vi "Check Error Status.vi"(0 "Emergency Stop":bool, 2 "Action (Write)":enum16{"Write", "Read"}(ring), 7 "Error In":errorcluster) -> (8 "Error?":bool)   [LabVIEW 2010]
doc: "This VI is a functional global variable. It checks for errors & remembers if one occurred. This is extremely useful between multiple loops. Be sure to initialize this VI before doing anything else."
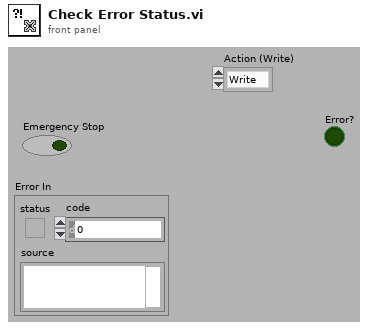
[diagram p1: front panel]
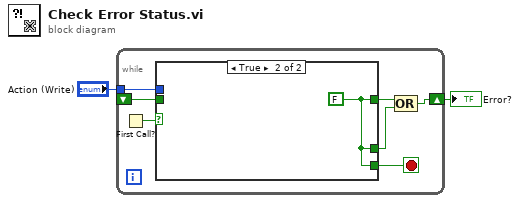
[diagram p0: block diagram]
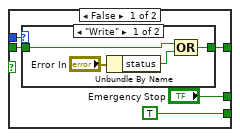
[diagram p2: hidden frame]
diagram:
  n1 = while {
    shift-right: [w5] -> w1
    shift-left: _ -> [w7]
    tunnel: "Action (Write)" -> [w8]
    stop <- w9 stop-if-true
    n2 = First Call?() -> (First Call?: T/F=w3:bool)
    n3 = case shown="TRUE" w3 {
      tunnel: [TRUE w20] -> w9
      tunnel: w8 -> [w13 _]
      tunnel: w7 -> [w12 _]
      tunnel: ["Emergency Stop" w20] -> w6
      tunnel: [w10 w20] -> w4
      frame False {
        n4 = case shown="\"Write\"" w13 {
          tunnel: [w15 w19] -> w10
          tunnel: w12 -> [w17 w19]
          frame "Write" {
            n5 = Unbundle By Name("Error In") -> ("status"=w16:bool)
            n6 = Compound Arithmetic op=OR(w17, w16) -> (w15:bool)
          }
          frame "Read" {
          }
        }
      }
      frame True {
        w20 = FALSE ("status")
      }
    }
    n7 = Compound Arithmetic op=OR(w4, w6) -> (w5:bool)
  }
  "Error?" <- w1
